vi "ActiveArray.vi"() -> ()   [LabVIEW 2020]
panel:
  out "Active":bool[](array[boolean])
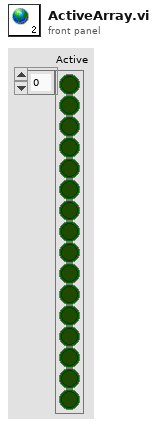
[diagram p1: front panel]
diagram:
